vi "SimpleAngleDifference.vi"(9 "Report in degrees? (False = Radians, default = True)":bool=TRUE, 10 "Angle 2":dbl, 11 "Angle 1":dbl) -> (2 "Absolute Difference":dbl, 3 "Difference":dbl)   [LabVIEW 2013]
doc: "Returns the angle between to headings, accounting for wraparound (0 and 355 are 5 degrees apart)\nCopied over from trunk."
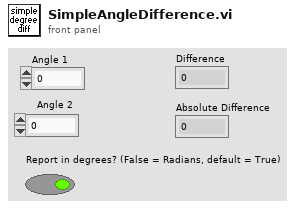
[diagram p1: front panel]
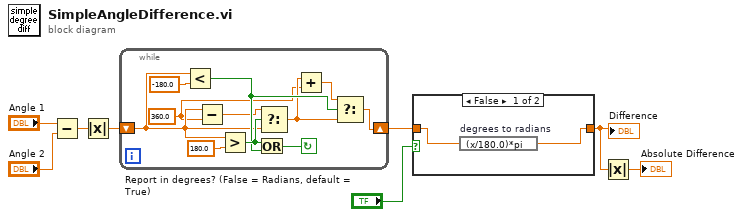
[diagram p0: block diagram]
diagram:
  n1 = Subtract(x="Angle 1", y="Angle 2") -> (x-y=w6:dbl)
  n2 = Absolute Value(x=w6) -> (abs(x)=w5:dbl)
  n3 = while {
    shift-right: [w9] -> w4
    shift-left: w5 -> [w14]
    stop <- w17 continue-if-true
    w12 = 360.0 ("y")
    n4 = Less?(x=w14, y=-180.0) -> (x < y?=w15:bool)
    n5 = Subtract(x=w14, y=w12) -> (x-y=w11:dbl)
    n6 = Greater?(x=w14, y=180.0) -> (0:w16:bool)
    n7 = Or(x=w16, y=w15) -> (x .or. y?=w17:bool)
    n8 = Select(t=w11, s=w16, f=w14) -> (s? t:f=w13:dbl)
    n9 = Add(x=w13, y=w12) -> (x+y=w10:dbl)
    n10 = Select(t=w10, s=w15, f=w13) -> (s? t:f=w9:dbl)
  }
  n11 = case shown="False" "Report in degrees? (False = Radians, default = True)" {
    tunnel: w4 -> [w21 w22]
    tunnel: [w20 w22] -> w2
    frame False {
      n12 = expression code="(x/180.0)*pi" "degrees to radians"(w21) -> (w20:dbl)
    }
    frame True {
    }
  }
  "Difference" <- w2
  n13 = Absolute Value(x=w2) -> (abs(x)=→"Absolute Difference":dbl)
